vi "AB_API Add Source Item.vi"(7 "top tree? (true)":bool=TRUE, 8 "error in":errorcluster, 9 "Source in":refnum<class "AB_Source.lvclass">, 10 "source items":refnum<class "AB_Source.lvclass">[](array[class]), 11 "Build in":refnum<class "AB_Build.lvclass">) -> (0 "error out":errorcluster, 3 "Build out":refnum<class "AB_Build.lvclass">)   [LabVIEW 2020]
uses:
  <vilib>/AppBuilder/AB_Classes/Source/AB_Source.lvclass
  <vilib>/AppBuilder/AB_Classes/Build/AB_Build.lvclass
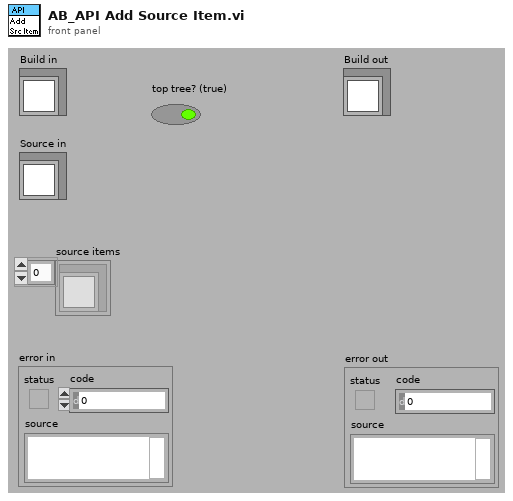
[diagram p1: front panel]
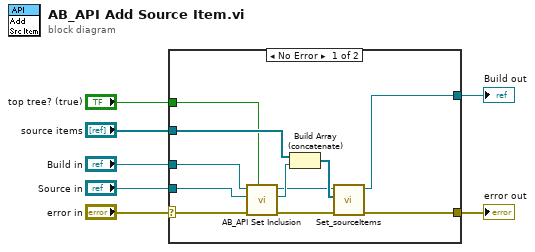
[diagram p0: block diagram]
diagram:
  n1 = case shown="No Error" "error in" {
    selector: "error in" -> [w13 w20]
    tunnel: "Source in" -> [w18 _]
    tunnel: "Build in" -> [w17 w19]
    tunnel: "source items" -> [w16 _]
    tunnel: [w15 w20] -> w4
    tunnel: [w14 w19] -> w3
    tunnel: "top tree? (true)" -> [w8 _]
    frame No Error {
      n2 = call <vilib>:"AB_API Set Inclusion.vi"("top tree? (true)"=w8, "error in (no error)"=w13, "Source in"=w18, "Build in"=w17) -> ("error out"=w10:errorcluster, "AB_Source_VI out"=w11:refnum<class "AB_Source.lvclass">, "AB_Build out"=w9:refnum<class "AB_Build.lvclass">)  [unwired: 5 in]
      n3 = Build Array (concatenate)(w16, w11) -> (w12:refnum<class "AB_Source.lvclass">[])
      n4 = call <vilib>:"Set_sourceItems.vi"("error in (no error)"=w10, "sourceItems"=w12, "Class in"=w9) -> ("error out"=w15:errorcluster, "Class out"=w14:refnum<class "AB_Build.lvclass">)  [unwired: 7 out]
    }
    frame Error {
    }
  }
  "error out" <- w4
  "Build out" <- w3
